vi "CURVA TEÓRICA RPS.vi"(0 "Resolución":dbl=1000.0, 1 "l(angstroms)":dbl=6328.0, 2 "Índices de refracción":refnum<vi>, 3 "q mínimo":dbl=30.0, 4 "q máximo":dbl=89.0, 5 "Número de capas":u32=1, 6 "Índices de refracción":dbl[](array[slide]) scale=0.0..10.0, 7 "Coeficientes de extinción":dbl[](array[slide]) scale=0.0..10.0, 8 "Coeficientes de extinción":refnum<vi>, 9 "Espesores":refnum<vi>, 10 "Espesores (angstroms)":dbl[](array[slide]) scale=0.0..1000.0, 11 "error in (no error)":errorcluster) -> (14 "EJE X":dbl[](array[numeric]), 15 "EJE Y TEÓRICO":dbl[](array[numeric]), 17 "q RPS teórico":dbl, 19 "error out":errorcluster)   [LabVIEW 2025]
panel:
  out "Curva RPS":cluster{"q0r":dbl[], dbl[]}(graph)
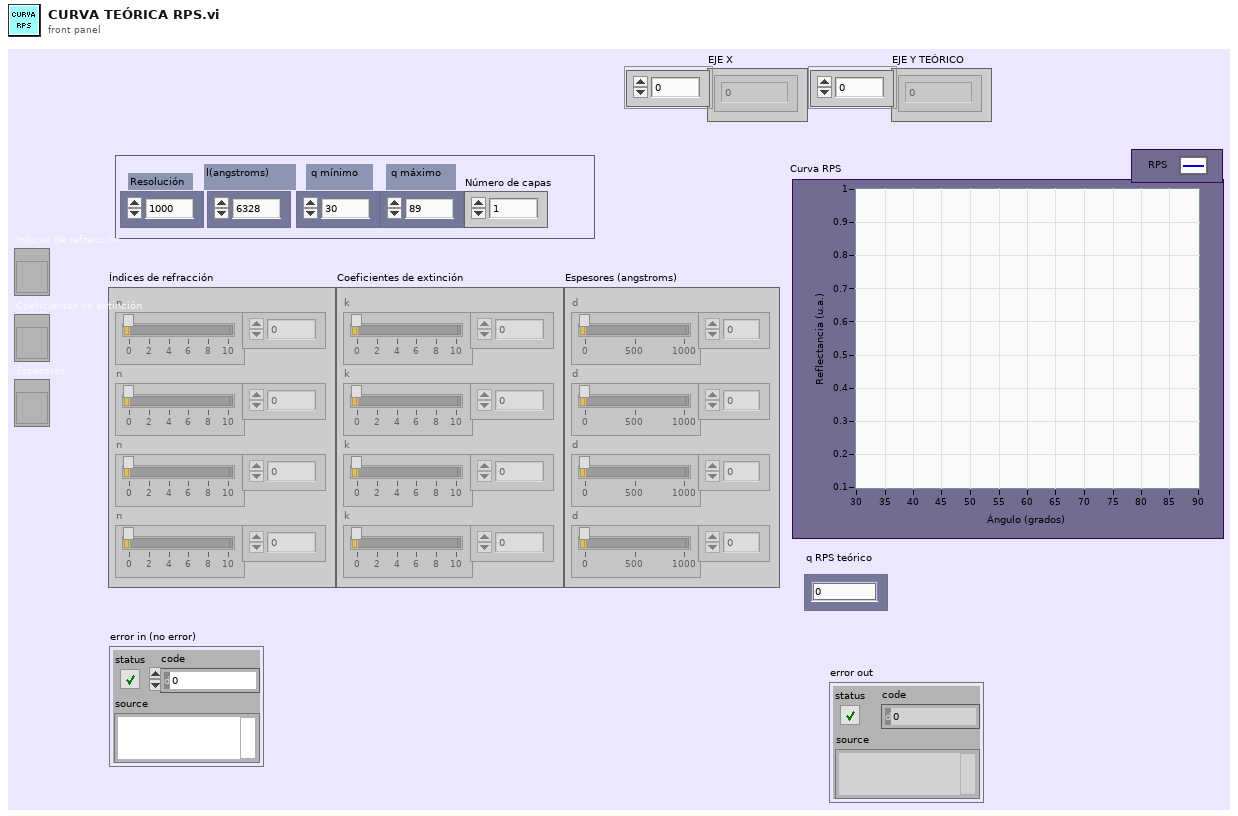
[diagram p1: front panel]
types:
  T1 = typedef "NI_Matrix.lvlib/ComplexMatrix.ctl" = cdb[][]
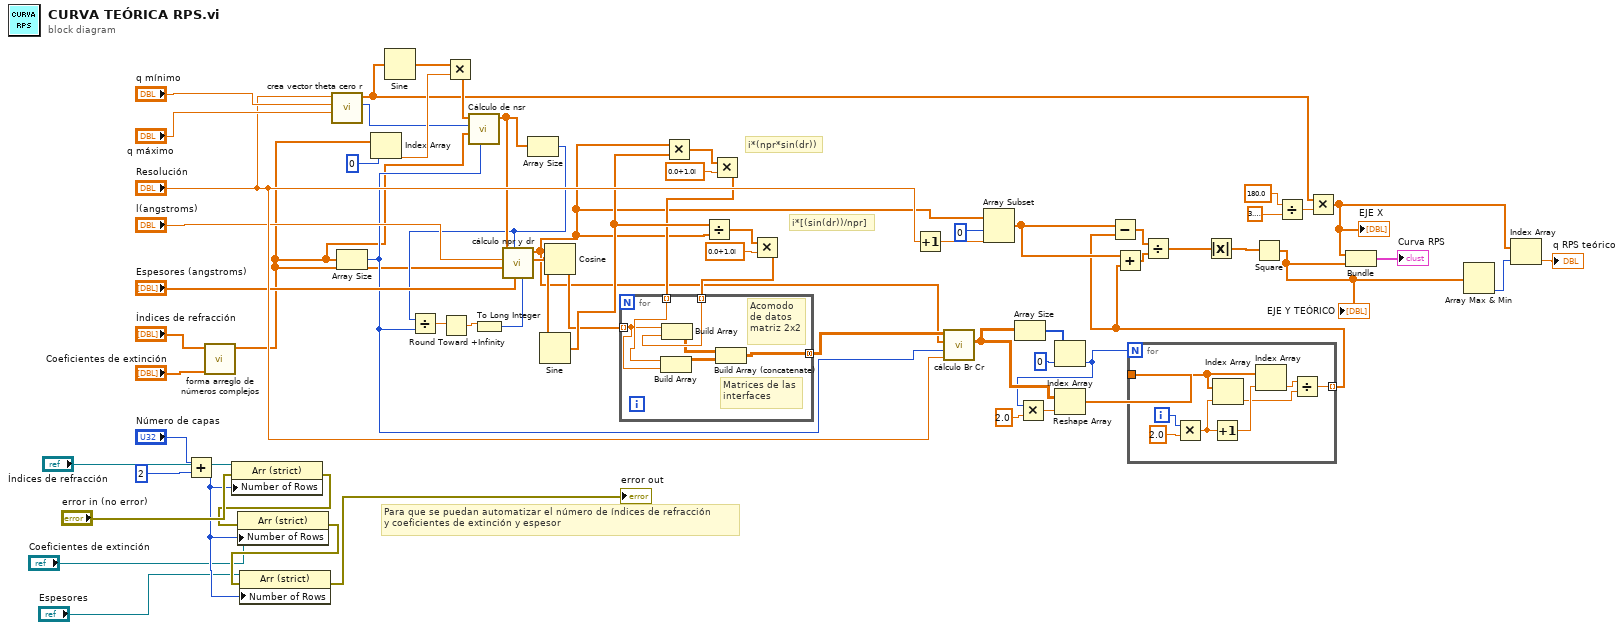
[diagram p0: block diagram]
diagram:
  # "i*[(sin(dr))/npr]"
  # "i*(npr*sin(dr))"
  # "Para que se puedan automatizar el número de índices de refracción\ny coeficientes de extinción y espesor"
  n1 = Add(x="Número de capas", y=u32 2) -> (x+y=w4:u32)
  n2 = call "forma arreglo de números complejos.vi"("Coeficientes de extinción"="Coeficientes de extinción", "Índices de refracción"="Índices de refracción") -> ("n + ik"=w12:cdb[])  [unwired: 9 in]
  n3 = property class="Arr (strict)"(reference="Índices de refracción", error in="error in (no error)", "Number of Rows"=w4) -> (error out=w7:errorcluster)  [unwired: 1 out]
  n4 = property class="Arr (strict)"(reference="Coeficientes de extinción", error in=w7, "Number of Rows"=w4) -> (error out=w6:errorcluster)  [unwired: 1 out]
  n5 = property class="Arr (strict)"(reference="Espesores", error in=w6, "Number of Rows"=w4) -> (error out=→"error out":errorcluster)  [unwired: 1 out]
  n6 = call "crea vector theta cero r.vi"("q máximo"="q máximo", "q mínimo"="q mínimo", "Resolución"="Resolución") -> ("Tamaño (r)"=w50:i32, "q0r"=w15:dbl[])  [unwired: 6 in, 1 out]
  n7 = Array Size(array=w12) -> (size(s)=w34:i32)
  n8 = Index Array(array=w12, index=0) -> (element=w51:cdb)
  n9 = Sine(x=w15) -> (sin(x)=w52:dbl[])
  n10 = Multiply(x=w52, y=w51) -> (x*y=w49:cdb[])
  n11 = call "Cálculo de nsr.vi"(">>tn>>"=w34, ">>n[]>>"=w12, "Tamaño (r)"=w50, ">>sr>>"=w49) -> (">>nsr>>"=w48:cdb[])  [unwired: 7 in]
  n12 = Array Size(array=w48) -> (size(s)=w36:i32)
  n13 = Divide(x=w36, y=w34) -> (x/y=w47:dbl)
  n14 = Round Toward +Infinity(x=w47) -> (ceil(x): smallest int >= x=w46:dbl)
  n15 = To Long Integer(number=w46) -> (32bit integer=w14:i32)
  n16 = call "cálculo npr y dr.vi"("Numeric Control"=w14, ">>d>>"="Espesores (angstroms)", "Numeric Control 2"=w36, ">>n[]>>"=w12, ">>lambda>>"="l(angstroms)", ">>nsr>>"=w48) -> (">>dr>>"=w45:cdb[], ">>nPr>>"=w26:csg[])  [unwired: 4 in]
  n17 = Sine(x=w45) -> (sin(x)=w42:cdb[])
  n18 = Cosine(x=w45) -> (cos(x)=w39:cdb[])
  n19 = Multiply(x=w26, y=w42) -> (x*y=w44:cdb[])
  n20 = Divide(x=w42, y=w26) -> (x/y=w41:cdb[])
  n21 = Multiply(x=w44, y=csg 0.0+1.0i) -> (x*y=w37:cdb[])
  n22 = Multiply(x=w41, y=csg 0.0+1.0i) -> (x*y=w38:cdb[])
  n23 = for {
    tunnel: [w70] -> w35 mode=concatenating
    tunnel: w39 -> [w67] mode=indexing
    tunnel: w38 -> [w69] mode=indexing
    tunnel: w37 -> [w68] mode=indexing
    # "Matrices de las\ninterfaces"
    # "Acomodo\nde datos\nmatriz 2x2"
    n24 = Build Array(w68, w67) -> (w65:T1)
    n25 = Build Array(w67, w69) -> (w66:T1)
    n26 = Build Array (concatenate)(w66, w65) -> (w70:T1)
  }
  n27 = Increment(x="Resolución") -> (x+1=w24:dbl)
  n28 = call "cálculo Br Cr.vi"("Resolución"="Resolución", "Número de índices de refracción"=w34, "npr"=w26, "Matrices interfaces"=w35) -> ("Br\nCr"=w33:cdb[][][])  [unwired: 4 in, 3 out]
  n29 = Array Subset(array=w26, index=0, length=w24) -> (w23:csg[])
  n30 = Array Size(array=w33) -> (size(s)=w32:i32[])
  n31 = Index Array(array=w32, index=0) -> (element=w27:i32)
  n32 = Multiply(x=w27, y=2.0) -> (x*y=w28:dbl)
  n33 = Reshape Array(w33, w28) -> (w29:cdb[])
  n34 = for {
    N: w27 -> [_]
    tunnel: w29 -> [w76]
    tunnel: [w71] -> w11 mode=indexing
    i -> [w77]
    n35 = Multiply(x=w77, y=2.0) -> (x*y=w75:dbl)
    n36 = Increment(x=w75) -> (x+1=w74:dbl)
    n37 = Index Array(array=w76, index=w75) -> (element=w72:cdb)
    n38 = Index Array(array=w76, index=w74) -> (element=w73:cdb)
    n39 = Divide(x=w73, y=w72) -> (x/y=w71:cdb)
  }
  n40 = Subtract(x=w23, y=w11) -> (x-y=w22:cdb[])
  n41 = Add(x=w23, y=w11) -> (x+y=w21:cdb[])
  n42 = Divide(x=w22, y=w21) -> (x/y=w20:cdb[])
  n43 = Absolute Value(x=w20) -> (abs(x)=w19:dbl[])
  n44 = Square(x=w19) -> (x^2=w54:dbl[])
  "EJE Y TEÓRICO" <- w54
  n45 = Divide(x=180.0, y=3.141592653589793) -> (x/y=w16:dbl)
  n46 = Multiply(x=w15, y=w16) -> (x*y=w55:dbl[])
  "EJE X" <- w55
  n47 = Bundle(w55, w54) -> (→"Curva RPS":cluster{dbl[], dbl[]})  [unwired: 1 in]
  n48 = Array Max & Min(array=w54) -> (min index (indices)=w13:i32)  [unwired: 3 out]
  n49 = Index Array(array=w55, index=w13) -> (element=→"q RPS teórico":dbl)
